vi "Initialization VI.vi"(8 "error in (no error)":errorcluster, 10 "Custom XML":string, 11 "Device Item Ref in":T1 format="%.0x") -> (0 "error out":errorcluster, 3 "Device Item Ref out":T1 format="%.0x")   [LabVIEW 2019, in "Control Addon System Explorer.lvlib"]
uses:
  Control Addon System Explorer.lvlib
  <vilib>/NI VeriStand/Custom Device API/Custom Device Item Ref.ctl
  <vilib>/NI/NI VeriStand Custom Device Import and Export Tool/ImportExport.lvlib
  Addon Shared/Control Addon Shared.lvlib
  <vilib>/NI VeriStand/Custom Device API/Custom Device API.lvlib
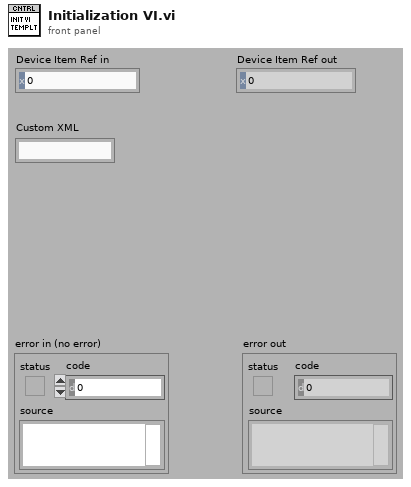
[diagram p1: front panel]
types:
  T1 = typedef "Custom Device API.lvlib/Custom Device Item Ref.ctl" = u64
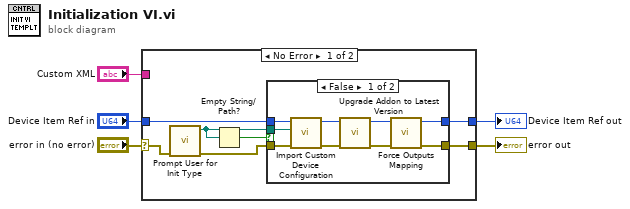
[diagram p0: block diagram]
diagram:
  n1 = case shown="No Error" "error in (no error)" {
    selector: "error in (no error)" -> [w9 w25]
    tunnel: [w10 w25] -> w5
    tunnel: [w12 w24] -> w3
    tunnel: "Device Item Ref in" -> [w11 w24]
    tunnel: "Custom XML" -> [_ _]
    frame No Error {
      n2 = call "Prompt User for Init Type.vi"("error in (no error)"=w9) -> ("error out"=w8:errorcluster, "Path out"=w7:path)  [unwired: 9 in]
      n3 = Empty String/Path?(string/path=w7) -> (empty?=w6:bool)
      n4 = case shown="False" w6 {
        tunnel: [w17 w22] -> w12
        tunnel: w11 -> [w21 w22]
        tunnel: [w18 w23] -> w10
        tunnel: w8 -> [w20 w23]
        tunnel: w7 -> [w19 _]
        frame False {
          n5 = call <vilib>:"Import Custom Device Configuration.vi"("error in (no error)"=w20, "Path"=w19, "NodeID"=w21) -> ("error out"=w16:errorcluster, "NodeID out"=w14:u64)  [unwired: 6 in, 1 out]
          n6 = call "Upgrade Addon to Latest Version.vi"("error in (no error)"=w16, "Device Item Ref in in"=w14) -> ("error out"=w15:errorcluster, "Device Item Ref out"=w13:T1)  [unwired: 8 in]
          n7 = call "Force Outputs Mapping.vi"("error in (no error)"=w15, "Device Item Ref in"=w13) -> ("error out"=w18:errorcluster, "Device Item Ref out"=w17:T1)  [unwired: 8 in]
        }
        frame True {
        }
      }
    }
    frame Error {
    }
  }
  "error out" <- w5
  "Device Item Ref out" <- w3
